vi "ELVIS III v1.0 Data Queue Ref Manager.vi"(6 "Action":enum16{"Get", "Reset"}(ring), 7 "error in (no error)":errorcluster) -> (0 "error out":errorcluster, 3 "Queue out":refnum<queue>)   [LabVIEW 2021]
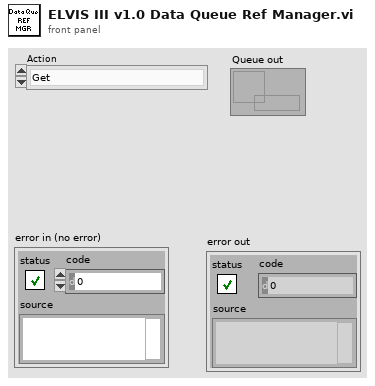
[diagram p1: front panel]
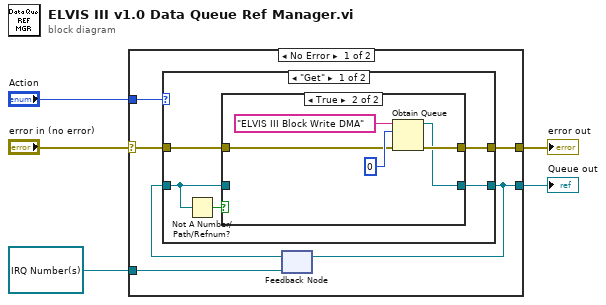
[diagram p0: block diagram]
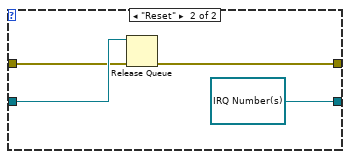
[diagram p3: hidden frame]
diagram:
  n1 = case shown="No Error" "error in (no error)" {
    selector: "error in (no error)" -> [w7 w28]
    tunnel: "Action" -> [w10 _]
    tunnel: refnum<queue> refnum ("queue out") -> [w9 w29]
    tunnel: [w8 w28] -> w4
    tunnel: [w6 w29] -> w2
    frame No Error {
      n2 = feedback #1(w9) -> (w11:refnum<queue>)
      n3 = case shown="\"Get\"" w10 {
        tunnel: w11 -> [w13 w26]
        tunnel: w7 -> [w15 w25]
        tunnel: [w14 w24] -> w8
        tunnel: [w12 refnum<queue> refnum ("queue out")] -> w6
        frame "Get" {
          n4 = Not A Number/Path/Refnum?(number/path/refnum=w13) -> (NaN/Path/Refnum?=w16:bool)
          n5 = case shown="True" w16 {
            tunnel: w15 -> [w17 w22]
            tunnel: [w17 w21] -> w14
            tunnel: [w18 w20] -> w12
            tunnel: w13 -> [w18 _]
            frame False {
            }
            frame True {
              n6 = Obtain Queue(name (unnamed)="ELVIS III Block Write DMA", element data type=0 ("IRQ Number(s)"), error in (no error)=w22) -> (queue out=w20:refnum<queue>, error out=w21:errorcluster)  [unwired: 2 in, 1 out]
            }
          }
        }
        frame "Reset" {
          n7 = Release Queue(queue=w26, error in (no error)=w25) -> (error out=w24:errorcluster)  [unwired: 1 in, 2 out]
        }
      }
      n8 = feedback-in #1(w6) -> ()
    }
    frame Error {
    }
  }
  "error out" <- w4
  "Queue out" <- w2
